vi "Set Generation Type.vi"(7 "Generation Type":T1, 8 "error in (no error)":errorcluster, 11 "Message in":T2 format="%.0x") -> (0 "error out":errorcluster, 3 "Message out":T2 format="%.0x")   [LabVIEW 2020, in "Instrument Addon Scripting API.lvlib"]
uses:
  Instrument Addon Scripting API.lvlib
  <vilib>/NI VeriStand/Custom Device API/Custom Device Item Ref.ctl
  Shared Directory/Message Generation Type.ctl
  Shared Directory/FG Control.ctl
  Shared Directory/Constants.vi
  <vilib>/NI VeriStand/Custom Device API/NI VeriStand - Get Item Property.vi
  <vilib>/NI VeriStand/Custom Device API/Get Item Property (U32).vi
  <vilib>/NI VeriStand/Custom Device API/Get Item Property (Double).vi
  <vilib>/NI VeriStand/Custom Device API/Get Item Property (Boolean).vi
  <vilib>/NI VeriStand/Custom Device API/Get Item Property (String).vi
  <vilib>/NI VeriStand/Custom Device API/NI VeriStand - Set Item Property.vi
  <vilib>/NI VeriStand/Custom Device API/Set Item Property (U32).vi
  <vilib>/NI VeriStand/Custom Device API/Set Item Property (Double).vi
  <vilib>/NI VeriStand/Custom Device API/Set Item Property (Boolean).vi
  <vilib>/NI VeriStand/Custom Device API/Set Item Property (String).vi
  Shared Directory/Instrument Addon Shared.lvlib
  <vilib>/NI VeriStand/Custom Device API/Custom Device API.lvlib
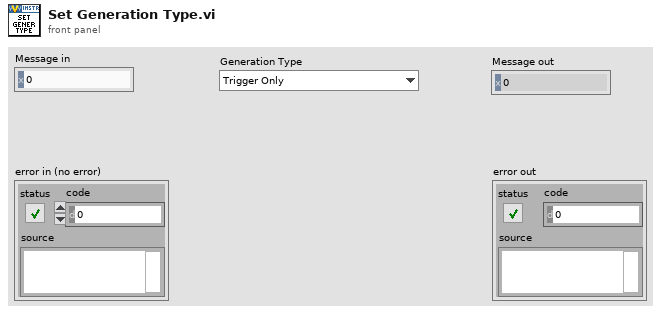
[diagram p1: front panel]
types:
  T1 = typedef "Instrument Addon Shared.lvlib/Message Generation Type.ctl" = enum16{"Trigger Only", "Periodic & Trigger", "Value Change & Trigger"}
  T2 = typedef "Custom Device API.lvlib/Custom Device Item Ref.ctl" = u64
  T3 = typedef "Instrument Addon Shared.lvlib/FG Control.ctl" = enum16{"Get", "Set"}
  T4 = typedef "Instrument Addon Shared.lvlib/Message Parameters.ctl" = cluster{"Generation Type":T1, "Period":dbl, "Include Protection":bool, "Type":string}
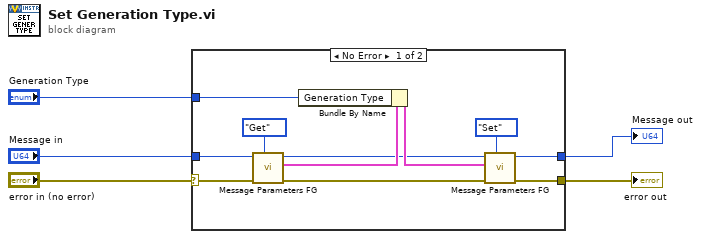
[diagram p0: block diagram]
diagram:
  n1 = case shown="No Error" "error in (no error)" {
    selector: "error in (no error)" -> [w6 w18]
    tunnel: [w16 w17] -> w5
    tunnel: [w15 w18] -> w4
    tunnel: "Message in" -> [w14 w17]
    tunnel: "Generation Type" -> [w13 _]
    frame No Error {
      n2 = call "Message Parameters FG.vi"("Action"=FG_Control."Get", "error in (no error)"=w6, "Item Ref in"=w14) -> ("error out"=w7:errorcluster, "Message Settings out"=w10:T4, "Item Ref out"=w8:T2)  [unwired: 6 in]
      n3 = Bundle By Name(cluster=w10, "Generation Type"=w13) -> (w11:T4)
      n4 = call "Message Parameters FG.vi"("Action"=FG_Control."Set", "error in (no error)"=w7, "Message Settings"=w11, "Item Ref in"=w8) -> ("error out"=w15:errorcluster, "Item Ref out"=w16:T2)  [unwired: 5 in, 1 out]
    }
    frame Error {
    }
  }
  "Message out" <- w5
  "error out" <- w4
